vi "CRC5 USB.vi"(5 "data":string) -> (2 "crc":string)   [LabVIEW 2021]
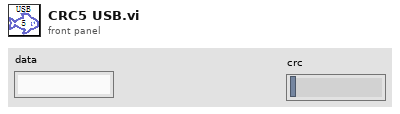
[diagram p1: front panel]
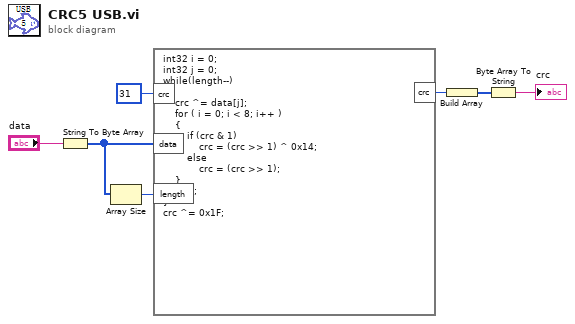
[diagram p0: block diagram]
diagram:
  n1 = String To Byte Array(string="data") -> (unsigned byte array=w6:u8[])
  n2 = Array Size(array=w6) -> (size(s)=w5:i32)
  n3 = formula code="int32 i = 0;\nint32 j = 0;\nwhile(length--)\n{\n    crc ^= data[j]; \n    for ( i = 0; i < 8; i++ )\n    {\n        if (crc & 1)\n            crc = (crc >> 1) ^ 0x14;\n        else\n            crc = (crc >> 1);\n    }\n    j++;\n}\ncrc ^= 0x1F;"("data"=w6, "length"=w5, "crc"=u8 31) -> ("crc"=w3:u8)
  n4 = Build Array(w3) -> (w2:u8[])
  n5 = Byte Array To String(unsigned byte array=w2) -> (string=→"crc":string)
